vi "xy_weight_height.vi"() -> ()   [LabVIEW 2022 SP3]
uses:
  <vilib>/Utility/file.llb/Read Delimited Spreadsheet (string).vi
panel:
  out "XY Graph":T1(graph)
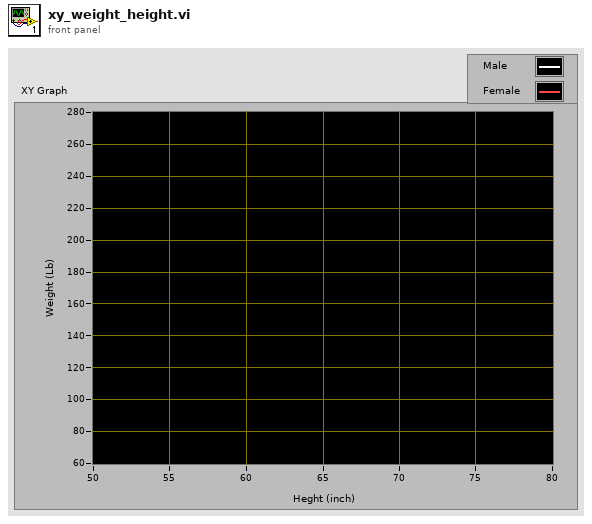
[diagram p1: front panel]
types:
  T1 = cluster{"female height":dbl[], "female weight":dbl[]}[]
  T2 = cluster{"female height":dbl[], "female weight":dbl[]}
  T3 = cluster{"male height":dbl[], "male weight":dbl[]}
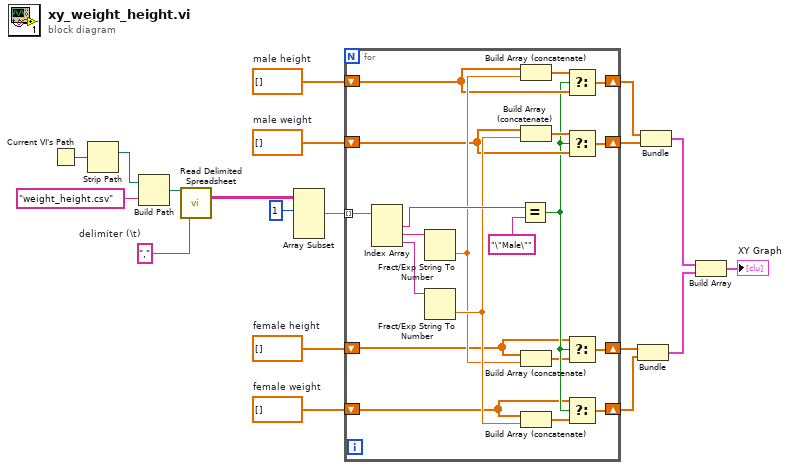
[diagram p0: block diagram]
diagram:
  w6 = dbl[] []  # female weight
  w7 = dbl[] []  # female height
  w10 = dbl[] []  # male weight
  w11 = dbl[] []  # male height
  w15 = ","  # delimiter (\t)
  n1 = Current VI's Path() -> (path=w19:path)
  n2 = Strip Path(path=w19) -> (stripped path=w18:path)  [unwired: 1 out]
  n3 = Build Path(base path=w18, name or relative path="weight_height.csv") -> (appended path=w16:path)
  n4 = call-poly <vilib>:"Read Delimited Spreadsheet.vi"("file path (dialog if empty)"=w16, "delimiter (\\t)"=w15) -> ("all rows"=w14:string[][])  [unwired: 8 in, 5 out]
  n5 = Array Subset(array=w14, index (row)=1 ("index")) -> (w12:string[][])  [unwired: 3 in]
  n6 = for {
    tunnel: w12 -> [w39] mode=indexing
    shift-right: [w34] -> w9
    shift-left: w11 -> [w28]
    shift-right: [w31] -> w8
    shift-left: w10 -> [w27]
    shift-right: [w20] -> w5
    shift-left: w7 -> [w25]
    shift-right: [w21] -> w4
    shift-left: w6 -> [w24]
    n7 = Index Array(array=w39) -> (element #1=w38:string, element #2=w36:string, element #3=w32:string)  [unwired: 3 in]
    n8 = Fract/Exp String To Number(string=w36) -> (number=w29:dbl)  [unwired: 3 in, 1 out]
    n9 = Fract/Exp String To Number(string=w32) -> (number=w30:dbl)  [unwired: 3 in, 1 out]
    n10 = Equal?(x=w38, y="\"Male\"") -> (x = y?=w26:bool)
    n11 = Build Array (concatenate)(w28, w29) -> (w35:dbl[])
    n12 = Build Array (concatenate)(w27, w30) -> (w33:dbl[])
    n13 = Build Array (concatenate)(w25, w29) -> (w23:dbl[])
    n14 = Build Array (concatenate)(w24, w30) -> (w22:dbl[])
    n15 = Select(t=w35, s=w26, f=w28) -> (s? t:f=w34:dbl[])
    n16 = Select(t=w33, s=w26, f=w27) -> (s? t:f=w31:dbl[])
    n17 = Select(t=w25, s=w26, f=w23) -> (s? t:f=w20:dbl[])
    n18 = Select(t=w24, s=w26, f=w22) -> (s? t:f=w21:dbl[])
  }
  n19 = Bundle("female height"=w5, "female weight"=w4) -> (w3:T2)  [unwired: 1 in]
  n20 = Bundle("male height"=w9, "male weight"=w8) -> (w2:T3)  [unwired: 1 in]
  n21 = Build Array(w2, w3) -> (→"XY Graph":T1)
